vi "LIDARRangingPose.vi"(8 "Previous X Position (in)":dbl, 9 "Distance to Target (in)":dbl, 10 "Heading to Target (deg)":dbl, 11 "Previous Y Position (in)":dbl) -> (1 "Delta Y (in)":dbl, 2 "Delta X (in)":dbl)   [LabVIEW 2019]
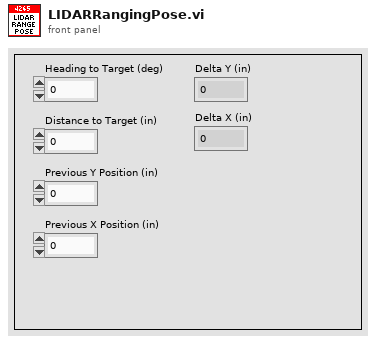
[diagram p1: front panel]
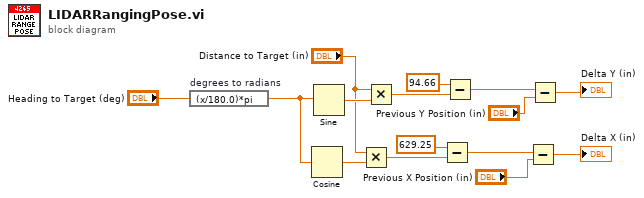
[diagram p0: block diagram]
diagram:
  n1 = expression code="(x/180.0)*pi" "degrees to radians"("Heading to Target (deg)") -> (w14:dbl)
  n2 = Cosine(x=w14) -> (cos(x)=w12:dbl)
  n3 = Sine(x=w14) -> (sin(x)=w13:dbl)
  n4 = Multiply(x="Distance to Target (in)", y=w12) -> (x*y=w7:dbl)
  n5 = Multiply(x="Distance to Target (in)", y=w13) -> (x*y=w9:dbl)
  n6 = Subtract(x=629.25, y=w7) -> (x-y=w3:dbl)
  n7 = Subtract(x=94.66, y=w9) -> (x-y=w6:dbl)
  n8 = Subtract(x=w3, y="Previous X Position (in)") -> (x-y=→"Delta X (in)":dbl)
  n9 = Subtract(x=w6, y="Previous Y Position (in)") -> (x-y=→"Delta Y (in)":dbl)
